vi "Set Mathematic Function Number.vi"(8 "error in (no error)":errorcluster, 10 "Number of Math. channels (max 5)":i32=1 min=1 max=5, 11 "VISA resource name":refnum<visa-resource-name>) -> (0 "error out":errorcluster, 3 "VISA resource name out":refnum<visa-resource-name>)   [LabVIEW 2017, in "Sefram DAS220.lvlib"]
doc: "Set the number of mathematic calculations on the device."
uses:
  <instrlib>/Sefram DAS220/Sefram DAS220.lvlib
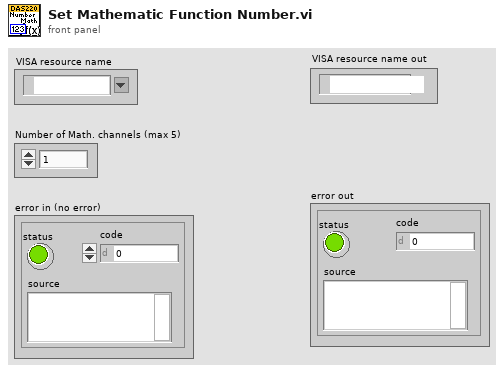
[diagram p1: front panel]
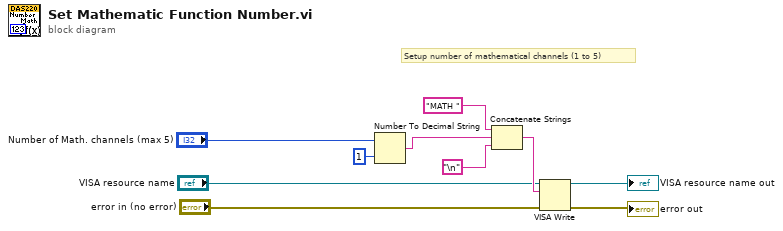
[diagram p0: block diagram]
diagram:
  # "Setup number of mathematical channels (1 to 5)"
  n1 = Number To Decimal String(number="Number of Math. channels (max 5)", width (-)=i16 1) -> (decimal integer string=w1:string)
  n2 = Concatenate Strings("MATH " ("string"), w1, "\n") -> (w10:string)
  n3 = VISA Write(VISA resource name="VISA resource name", write buffer=w10, error in (no error)="error in (no error)") -> (VISA resource name out=→"VISA resource name out":refnum<visa-resource-name>, error out=→"error out":errorcluster)  [unwired: 1 out]
